vi "Frame_to_word_15693 UP.vi"() -> ()   [LabVIEW 2019]
uses:
  <vilib>/express/express analysis/Spectral/Block/exnSpectralBlock spectral measurements RMS poly.vi
  <vilib>/express/express analysis/Spectral/Block/exnSpectralBlock spectral measurements RMS WFM.vi
  <vilib>/addons/Modulation/Analog/MT Modulate AM (DSB).vi
  <vilib>/addons/Modulation/Analog/MT Upconvert Baseband (Real).vi
  <vilib>/ErrorRing/Error Ring.xnode
  <vilib>/express/express analysis/Spectral/XNode/ExpressSpectralMeasurementsBlockNode.xnode
  <vilib>/addons/Modulation/niAMT.lvlib
panel:
  out "video Manchecter 8":cluster{"t0":dbl, "dt":dbl, "Y":dbl[]}(graph)
  out "video Manchecter 2":cluster{"t0":dbl, "dt":dbl, "Y":dbl[]}(graph)
  out "video Manchecter 7":waveform(dbl)(graph)
  out "video Manchecter 6":cluster{"t0":dbl, "dt":dbl, "Y":dbl[]}(graph)
  out "video Manchecter 5":waveform(dbl)(graph)
  out "video Manchecter 4":cluster{"t0":dbl, "dt":dbl, "Y":dbl[]}(graph)
  out "video Manchecter":cluster{"t0":dbl, "dt":dbl, "Y":dbl[]}(graph)
  in  "BIT RATE":dbl
  in  "CARRIER (hz)":dbl=13560.0
  out "Video  without CRC":cluster{"t0":dbl, "dt":dbl, "Y":dbl[]}(graph)
  out "Video":cluster{"t0":dbl, "dt":dbl, "Y":dbl[]}(graph)
  in  "Flag":u8[](array[numeric])=[210] format="%x"
  in  "UID":u8[](array[numeric])=[3, 241, 229, 208, 4, 255] format="%x"
  in  "DSFID":u8[](array[numeric])=[243] format="%x"
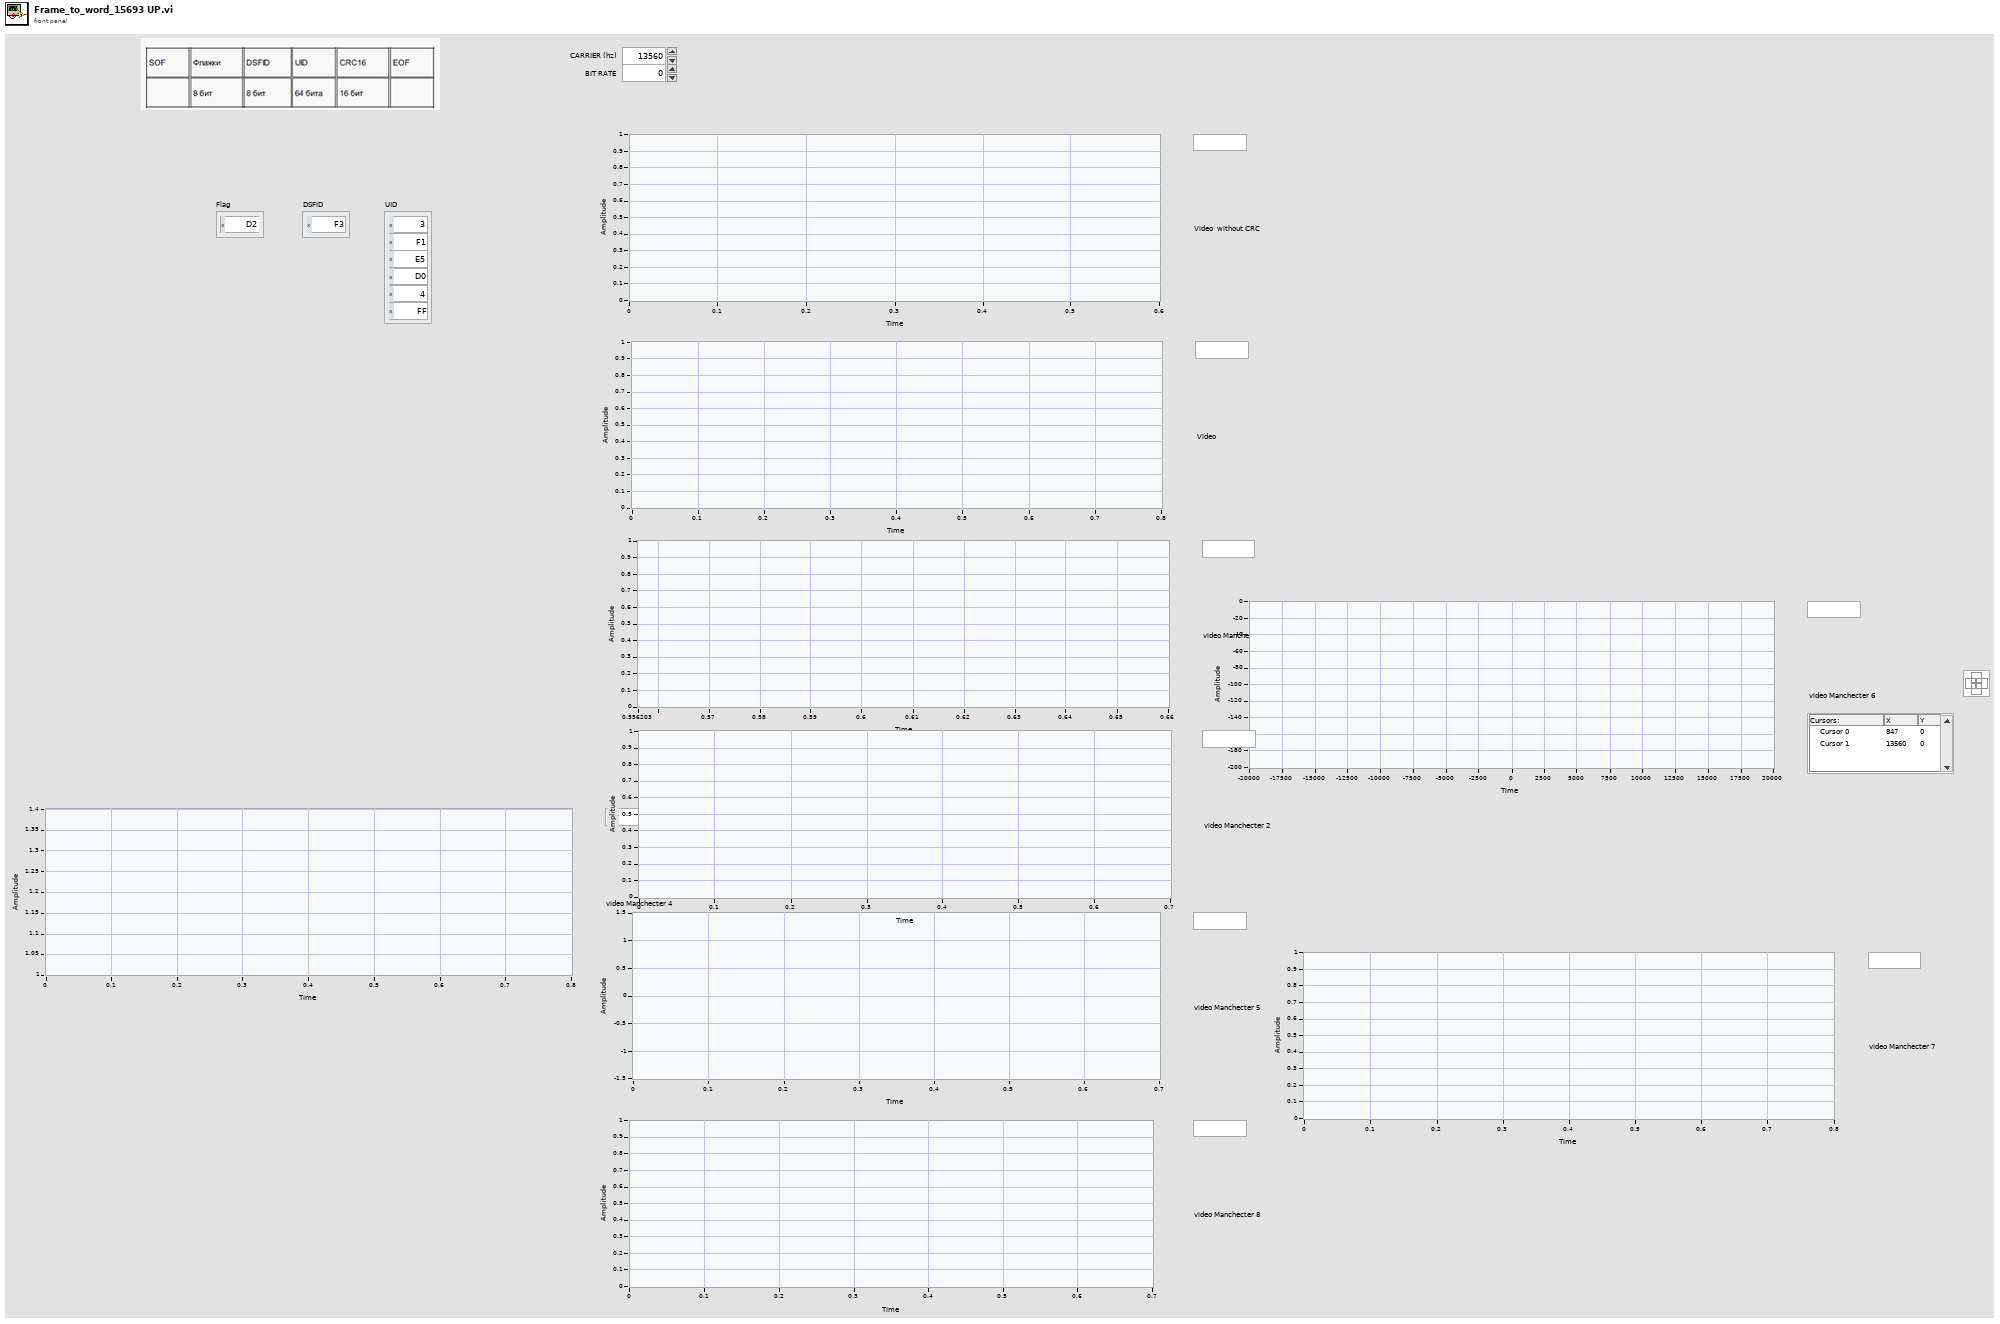
[diagram p1: front panel]
types:
  T1 = typedef "niAMT.lvlib/Complex Data Waveform.ctl" = cluster{"t0":dbl, "dt":dbl, "Y":cdb[]}
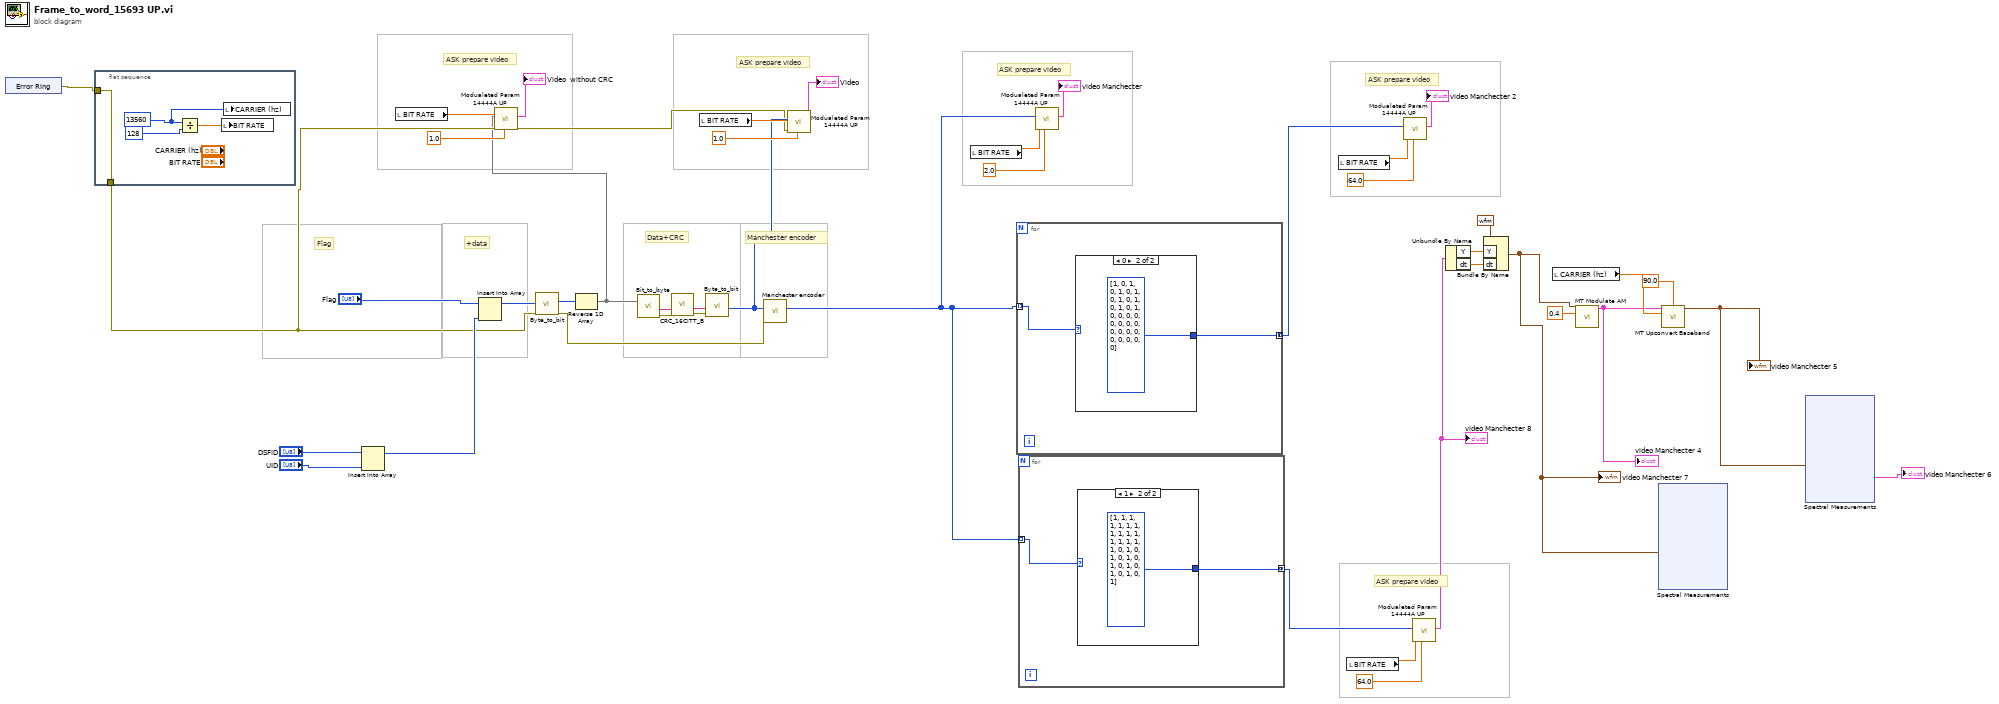
[diagram p0: block diagram]
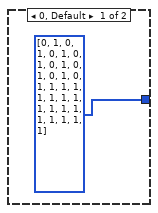
[diagram p2: hidden frame]
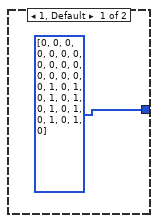
[diagram p3: hidden frame]
diagram:
  # "ASK prepare video"
  # "ASK prepare video"
  # "ASK prepare video"
  # "ASK prepare video"
  # "ASK prepare video"
  # "ASK prepare video"
  # "Manchester encoder"
  # "Data+CRC"
  # "+data"
  # "Flag"
  n1 = xnode "Error Ring"() -> ("error out"=w31:errorcluster)
  n2 = flat-sequence {
    tunnel: w31 -> [w45]
    tunnel: [w45] -> w30
    frame #0 {
      w46 = u32 13560
      n3 = Divide(x=w46, y=u32 128) -> (x/y=w47:dbl)
      n4 = local write "BIT RATE"(w47) -> ()
      n5 = local write "CARRIER (hz)"(w46) -> ()
    }
  }
  n6 = Insert Into Array(array="DSFID", new element="UID") -> (w42:u8[])  [unwired: 1 in]
  n7 = local read "BIT RATE"() -> (w36:dbl)
  n8 = Insert Into Array(array="Flag", new element=w42) -> (w34:u8[])  [unwired: 1 in]
  n9 = call "Byte_to_bit.vi"("Error In"=w30, "Array of byte"=w34) -> ("Error Out"=w32:errorcluster, "Arrray of bit"=w33:u8[])  [unwired: 5 in, 1 out]
  n10 = Reverse 1D Array(array=w33) -> (reversed array=w28:u8[])
  n11 = call "Modualeted Param 14444A UP.vi"("encoder divider"=1.0 ("y"), "Error In"=w30, "BIT RATE"=w36, "Bit stream out (NRZ encode)"=w28) -> ("Error Out"=w29:errorcluster, "output complex waveform"=→"Video  without CRC":T1)  [unwired: 6 in]
  n12 = call "Bit_to_byte.vi"("Array of bit"=w28) -> ("Error Out"=w4:errorcluster, "BYTE"=w2:string)  [unwired: 8 in, 1 out]
  n13 = call "CRC_16CITT_B.vi"("Error In"=w4, "DATA PACKET"=w2) -> ("Error Out"=w3:errorcluster, "DATA PACKET+CRC"=w1:string)  [unwired: 5 in, 1 out]
  n14 = local read "BIT RATE"() -> (w41:dbl)
  n15 = call "Byte_to_bit.vi"("Error In"=w3, "BYTE"=w1) -> ("Arrray of bit (str)"=w35:u8[])  [unwired: 5 in, 2 out]
  n16 = call "Manchester encoder.vi"("Error In"=w32, "Bit stream in"=w35) -> ("Bit stream out (Manchester encode)"=w12:u8[])  [unwired: 8 in, 1 out]
  n17 = call "Modualeted Param 14444A UP.vi"("encoder divider"=1.0 ("y"), "Error In"=w29, "BIT RATE"=w41, "Bit stream out (NRZ encode)"=w35) -> ("output complex waveform"=→"Video":T1)  [unwired: 6 in, 1 out]
  n18 = local read "BIT RATE"() -> (w26:dbl)
  n19 = for {
    tunnel: w12 -> [w50] mode=indexing
    tunnel: [w49] -> w22 mode=concatenating
    n20 = case shown="0" w50 {
      tunnel: [u8[] [0, 0, 0, 0, 0, 0, 0, 0, 0, 0, 0, 0, 0, 0, 0, 0, 1, 0, 1, 0, 1, 0, 1, 0, 1, 0, 1, 0, 1, 0, 1, 0] ("output array") u8[] [1, 0, 1, 0, 1, 0, 1, 0, 1, 0, 1, 0, 1, 0, 1, 0, 0, 0, 0, 0, 0, 0, 0, 0, 0, 0, 0, 0, 0, 0, 0, 0] ("output array")] -> w49
      frame 1, Default {
      }
      frame 0 {
      }
    }
  }
  n21 = for {
    tunnel: w12 -> [w54] mode=indexing
    tunnel: [w53] -> w9 mode=concatenating
    n22 = case shown="1" w54 {
      tunnel: [u8[] [0, 1, 0, 1, 0, 1, 0, 1, 0, 1, 0, 1, 0, 1, 0, 1, 1, 1, 1, 1, 1, 1, 1, 1, 1, 1, 1, 1, 1, 1, 1, 1] ("output array") u8[] [1, 1, 1, 1, 1, 1, 1, 1, 1, 1, 1, 1, 1, 1, 1, 1, 0, 1, 0, 1, 0, 1, 0, 1, 0, 1, 0, 1, 0, 1, 0, 1] ("output array")] -> w53
      frame 0, Default {
      }
      frame 1 {
      }
    }
  }
  n23 = call "Modualeted Param 14444A UP.vi"("encoder divider"=2.0 ("y"), "BIT RATE"=w26, "Bit stream out (NRZ encode)"=w12) -> ("output complex waveform"=→"video Manchecter":T1)  [unwired: 7 in, 1 out]
  n24 = local read "BIT RATE"() -> (w24:dbl)
  n25 = local read "BIT RATE"() -> (w11:dbl)
  n26 = call "Modualeted Param 14444A UP.vi"("encoder divider"=64.0 ("y"), "BIT RATE"=w24, "Bit stream out (NRZ encode)"=w22) -> ("output complex waveform"=→"video Manchecter 2":T1)  [unwired: 7 in, 1 out]
  n27 = call "Modualeted Param 14444A UP.vi"("encoder divider"=64.0 ("y"), "BIT RATE"=w11, "Bit stream out (NRZ encode)"=w9) -> ("output complex waveform"=w7:T1)  [unwired: 7 in, 1 out]
  "video Manchecter 8" <- w7
  n28 = Unbundle By Name(w7) -> ("Y"=w15:cdb[], "dt"=w14:dbl)
  n29 = Bundle By Name(cluster=waveform(cdb) {"t0"=timestamp(0 s since 1904-01-01), "dt"=1.0, "Y"=[]} ("waveform"), "Y"=w15, "dt"=w14) -> (w13:waveform(cdb))
  "video Manchecter 7" <- w13
  n30 = local read "CARRIER (hz)"() -> (w20:dbl)
  n31 = call-poly <vilib>:"MT Modulate AM.vi"("message signal"=w13, "modulation index"=0.4) -> ("AM modulated waveform"=w18:cluster{"t0":dbl, "dt":dbl, "Y":cdb[]})  [unwired: 12 in, 1 out]
  "video Manchecter 4" <- w18
  n32 = xnode "Spectral Measurements"("Signals"=w13) -> ()  [unwired: 1 in, 3 out]
  n33 = call-poly <vilib>:"MT Upconvert Baseband.vi"("baseband waveform (complex)"=w18, "initial phase (deg)"=90.0, "carrier frequency (Hz)"=w20) -> ("passband waveform"=w17:waveform(dbl))  [unwired: 11 in, 1 out]
  "video Manchecter 5" <- w17
  n34 = xnode "Spectral Measurements"("Signals"=w17) -> ("FFT - (RMS)"=→"video Manchecter 6":cluster{"f0":dbl, "df":dbl, "magnitude":dbl[]})  [unwired: 1 in, 2 out]
